vi "Set Body (XML).vi"(6 "charset (\"us-ascii\")":string="us-ascii", 8 "error in (no error)":errorcluster, 10 "Body":string, 11 "Response in":refnum<class "Response.lvclass">) -> (0 "error out":errorcluster, 3 "Response out":refnum<class "Response.lvclass">)   [LabVIEW 2023, in "Response.lvclass"]
uses:
  Response.lvclass
  Response.lvclass/Response.ctl
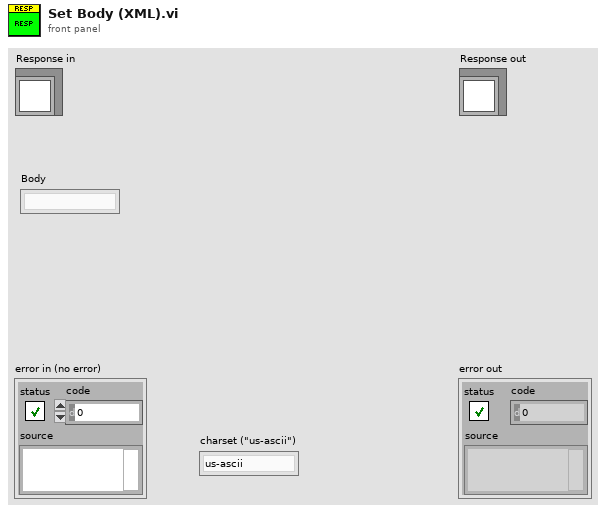
[diagram p1: front panel]
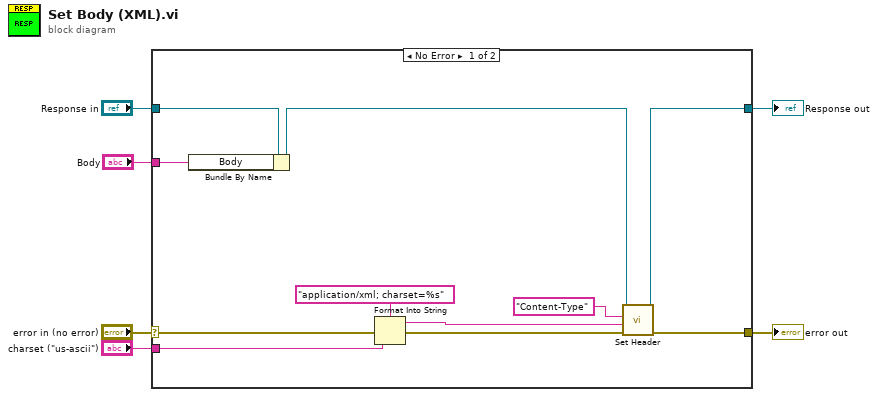
[diagram p0: block diagram]
diagram:
  n1 = case shown="No Error" "error in (no error)" {
    selector: "error in (no error)" -> [w15 w19]
    tunnel: [w12 w19] -> w5
    tunnel: [w11 w18] -> w3
    tunnel: "Response in" -> [w17 w18]
    tunnel: "Body" -> [w16 _]
    tunnel: "charset (\"us-ascii\")" -> [w9 _]
    frame No Error {
      n2 = Bundle By Name(cluster=w17, "Body"=w16) -> (w14:refnum<class "Response.lvclass">)
      n3 = Format Into String(format string="application/xml; charset=%s" ("Delimiter"), error in=w15, w9) -> (resulting string=w8:string, error out=w10:errorcluster)  [unwired: 1 in]
      n4 = call "Set Header.vi"("error in (no error)"=w10, "Value"=w8, "Header"="Content-Type" ("Delimiter"), "Response in"=w14) -> ("error out"=w12:errorcluster, "Response out"=w11:refnum<class "Response.lvclass">)  [unwired: 5 in, 1 out]
    }
    frame Error {
    }
  }
  "error out" <- w5
  "Response out" <- w3
